vi "MakeExample.vi"(8 "error in (no error)":errorcluster, 9 "TriggerRefractoryPeriod (Frames)":i32, 10 "StimulusObject Parameters":variant, 11 "StimulusObject in":refnum<class "StimulusObject.lvclass">) -> (0 "error out":errorcluster, 3 "StimulusObject out":refnum<class "StimulusObject.lvclass">)   [LabVIEW 2019, in "StimulusObject.lvclass"]
uses:
  StimulusObject.lvclass
  StimulusObject.lvclass/StimulusObject.ctl
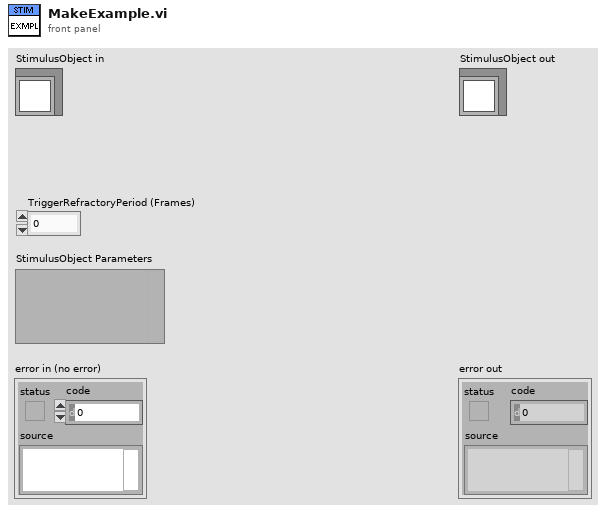
[diagram p1: front panel]
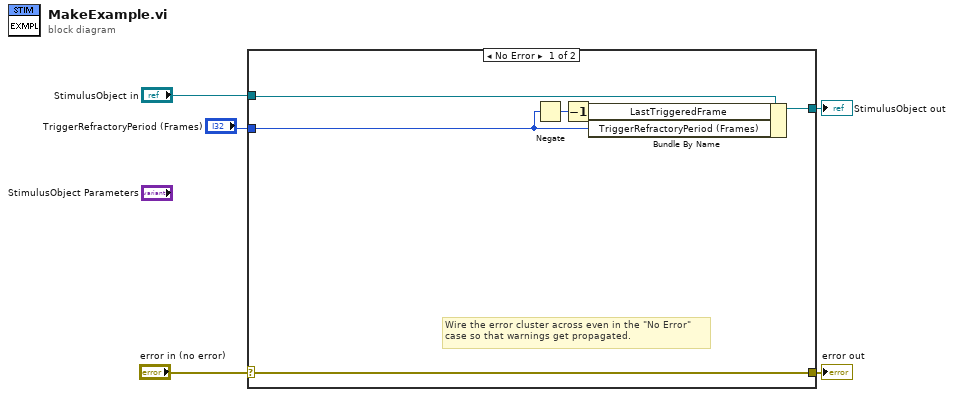
[diagram p0: block diagram]
diagram:
  n1 = case shown="No Error" "error in (no error)" {
    selector: "error in (no error)" -> [w11 w13]
    tunnel: [w11 w13] -> w4
    tunnel: [w9 w12] -> w2
    tunnel: "StimulusObject in" -> [w10 w12]
    tunnel: "TriggerRefractoryPeriod (Frames)" -> [w6 _]
    frame No Error {
      # "Wire the error cluster across even in the \"No Error\"\ncase so that warnings get propagated."
      n2 = Negate(x=w6) -> (-x=w7:i32)
      n3 = Decrement(x=w7) -> (x-1=w8:i32)
      n4 = Bundle By Name(cluster=w10, "LastTriggeredFrame"=w8, "TriggerRefractoryPeriod (Frames)"=w6) -> (w9:refnum<class "StimulusObject.lvclass">)
    }
    frame Error {
    }
  }
  "error out" <- w4
  "StimulusObject out" <- w2
